vi "convertRoleToFunction.vi"(8 "error in (no error)":errorcluster, 10 "role":T2=enum."DefenderArea", 11 "Game in":refnum<class "Game.lvclass">) -> (0 "error out":errorcluster, 2 "function":T1, 3 "Game out":refnum<class "Game.lvclass">)   [LabVIEW 2023, in "Game.lvclass"]
uses:
  Game.lvclass
  Robot_class/roles.ctl
  Vision_class/Old vision/Controls/Functions Enum.ctl
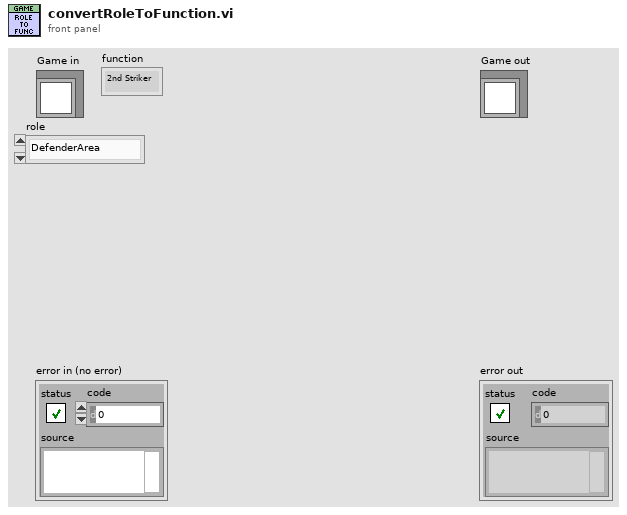
[diagram p1: front panel]
types:
  T1 = typedef "Functions Enum.ctl" = enum16{"2nd Striker", "Attacker", "Goalie", "Defender", "Striker", "Goto 0", "Dummy", "Kicker", "ZigZag 0", "ZigZag 1", "ZigZag 2", "ZigZag 3", "ZigZag 4", "ZigZag 5", "ZigZag 6", "ZigZag 7", "ZigZag 8", ""}
  T2 = typedef "roles.ctl" = enum16{"BallChallengerAttackerVSS", "NormalAttackerVSS", "AttackerAimGoalVSS", "DefenderAreaVSS", "KeeperVSS", "Tabler", "TableFinalizer", "PrepareRollToPassRoller", "PrepareRollToPassReceiver", "SimplePassRoll", "SimplePassRollReceiver", "PenaltyDefense", "PreparePassReceiver 2", "PreparePassReceiver 1", "PassObserver", "Timeout", "Goto", "ZigZag", "None", "BallOutOfField", "DefenderArea", "Duelist", "AttackerStop", "FollowAttacker", "KeeperRole", "KickPenalty", "AttackerAimGoal", "AttackerBlock", "Marker", "Halt", "Shoot", "PassKicker", "PassReceiver", "TestRole", "PenaltyAttacker"}
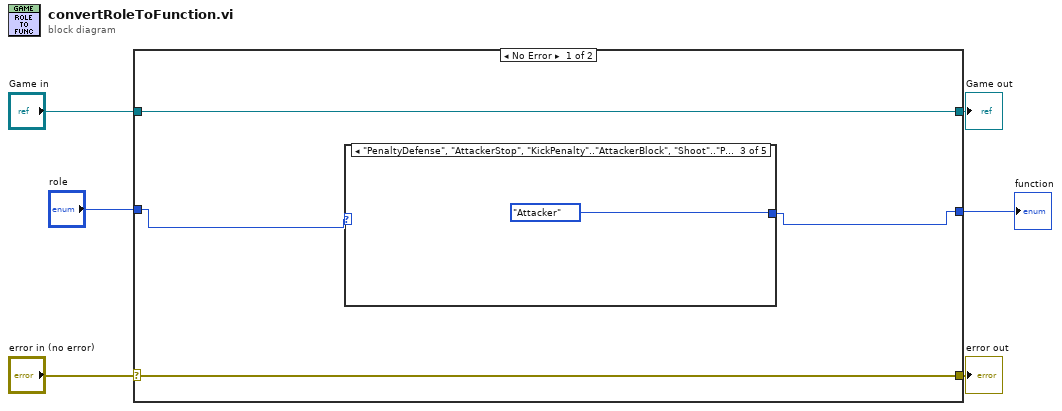
[diagram p0: block diagram]
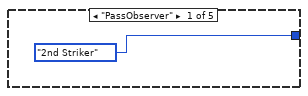
[diagram p2: hidden frame]
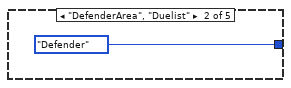
[diagram p3: hidden frame]
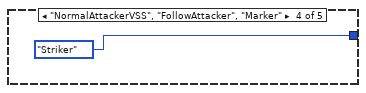
[diagram p4: hidden frame]
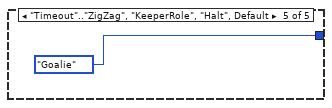
[diagram p5: hidden frame]
diagram:
  n1 = case shown="No Error" "error in (no error)" {
    selector: "error in (no error)" -> [w9 w17]
    tunnel: [w9 w17] -> w5
    tunnel: [w10 w16] -> w3
    tunnel: "Game in" -> [w10 w16]
    tunnel: "role" -> [w8 _]
    tunnel: [w7 _] -> w1
    frame No Error {
      n2 = case shown="\"PenaltyDefense\", \"AttackerStop\", \"KickPenalty\"..\"AttackerBlock\", \"Shoot\"..\"PassReceiver\", \"PenaltyAttacker\"" w8 {
        tunnel: [Functions_Enum."2nd Striker" ("function") Functions_Enum."Defender" ("function") Functions_Enum."Attacker" ("function") Functions_Enum."Striker" ("function") Functions_Enum."Goalie" ("function")] -> w7
        frame "PassObserver" {
        }
        frame "DefenderArea", "Duelist" {
        }
        frame "PenaltyDefense", "AttackerStop", "KickPenalty".."AttackerBlock", "Shoot".."PassReceiver", "PenaltyAttacker" {
        }
        frame "NormalAttackerVSS", "FollowAttacker", "Marker" {
        }
        frame "Timeout".."ZigZag", "KeeperRole", "Halt", Default {
        }
      }
    }
    frame Error {
    }
  }
  "error out" <- w5
  "Game out" <- w3
  "function" <- w1
